vi "Destructor__icon_lib_labview_project_api.vi"(7 "Close Project (F)":bool, 8 "error in (no error)":errorcluster, 9 "Save Path":path, 10 "Save Project (F)":bool, 11 "Project Reference":refnum<vi>) -> (0 "error out":errorcluster)   [LabVIEW 2016, in "LabVIEW Project API__icon_lib_labview_project_api.lvlib"]
doc: "Close a Project\n\n<b>Author:</b> JG\n\n<b>ICON Technologies Pty Ltd</b>\nCopyright (C) 1990-2009\nAll Rights Reserved"
uses:
  LabVIEW Project API__icon_lib_labview_project_api.lvlib
panel:
  # "Output"
  # "Input"
  # "ICON Technologies Pty Ltd\nCopyright (C) 1990-2009\nAll Rights Reserved"
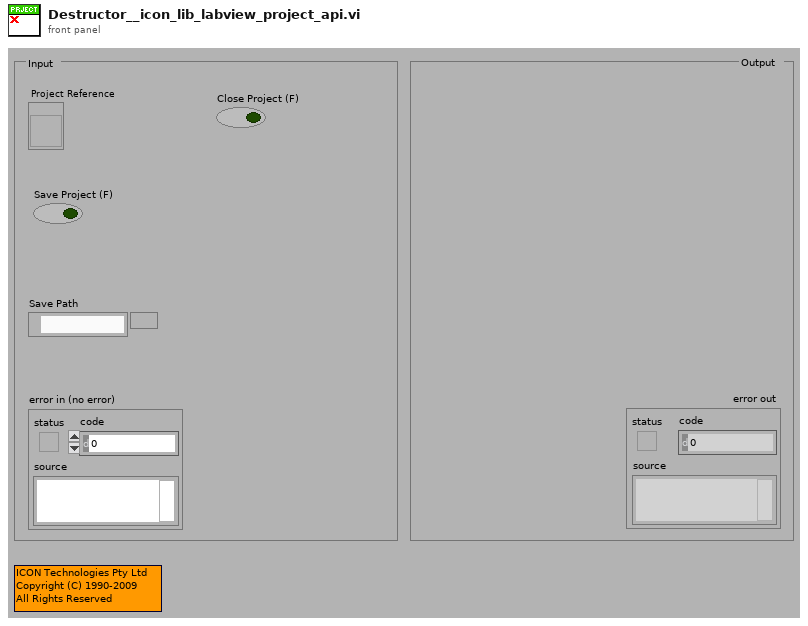
[diagram p1: front panel]
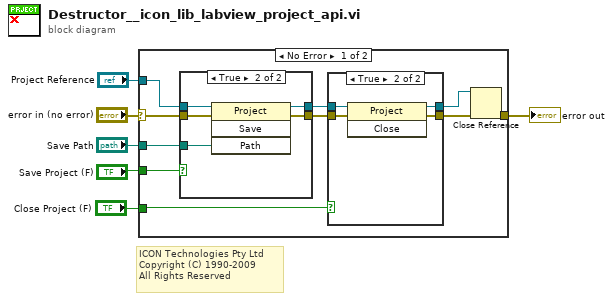
[diagram p0: block diagram]
diagram:
  # "ICON Technologies Pty Ltd\nCopyright (C) 1990-2009\nAll Rights Reserved"
  n1 = case shown="No Error" "error in (no error)" {
    selector: "error in (no error)" -> [w16 w30]
    tunnel: [w9 w30] -> w5
    tunnel: "Save Path" -> [w15 _]
    tunnel: "Project Reference" -> [w14 _]
    tunnel: "Save Project (F)" -> [w13 _]
    tunnel: "Close Project (F)" -> [w7 _]
    frame No Error {
      n2 = case shown="True" w13 {
        tunnel: w16 -> [w23 w29]
        tunnel: w15 -> [_ w28]
        tunnel: w14 -> [w24 w27]
        tunnel: [w23 w26] -> w11
        tunnel: [w24 w25] -> w12
        frame False {
        }
        frame True {
          n3 = invoke class="Project" method="Save"(reference=w27, error in=w29, "Path"=w28) -> (reference out=w25:refnum<vi>, error out=w26:errorcluster)  [unwired: 1 in, 2 out]
        }
      }
      n4 = case shown="True" w7 {
        tunnel: w12 -> [w18 w22]
        tunnel: w11 -> [w17 w21]
        tunnel: [w17 w20] -> w10
        tunnel: [w18 w19] -> w8
        frame False {
        }
        frame True {
          n5 = invoke class="Project" method="Close"(reference=w22, error in=w21) -> (reference out=w19:refnum<vi>, error out=w20:errorcluster)  [unwired: 1 in, 1 out]
        }
      }
      n6 = Close Reference(reference=w8, error in (no error)=w10) -> (error out=w9:errorcluster)
    }
    frame Error {
    }
  }
  "error out" <- w5
